vi "x410_test_fpga_with_ref.vi"() -> ()   [LabVIEW 2025]
doc: "this VI is the top level of the FPGA.\n\nsubVIs placed at this level:\nmust have fixed-sized arrays.\ncontaining a class input (control) must NOT be left unconnected.\n\nconditional symbols supported for ease-of-use in building variations of the image are documented in a comment section and should be kept up-to-date."
uses:
  <vilib>/Platform/TimedLoop/XDataNode/timing_clust.ctl
  <vilib>/Platform/TimedLoop/XDataNode/nitl_modes.ctl
  <vilib>/Platform/TimedLoop/XDataNode/wakeup.ctl
  Aqc_loop_states.ctl
  <vilib>/rvi/Emulation/niFpgaSctlEmulationGetInTimedLoop.vi
  <vilib>/rvi/Emulation/niFpgaEmulationReportErrorSimple.vi
  <vilib>/rvi/Emulation/niFpgaGetClockAttributes.vi
  <vilib>/rvi/Emulation/niFpgaCriticalErrorInLSC.vi
  <vilib>/rvi/Emulation/niFpgaProcessEmulError.vi
  <vilib>/rvi/interface/RandomDataEmulation/nirviRandomDataMultiElementFPGAFIFO.vi
  <instcachedir>/0/nirviRandomDataMultiElementFPGAFIFO_BE2FF10D3D6E420AB0291A02835C249E.lvgen/nirviRandomDataMultiElementFPGAFIFO_BE2FF10D3D6E420AB0291A02835C249E_001.vi
  <vilib>/rvi/interface/RandomDataEmulation/niFpgaRandomDataHandleErrors.vi
  <vilib>/Platform/TimedLoop/XDataNode/XDataNode.xnode
  <vilib>/rvi/DataTransferAndStorage/Container/XNode/niFpgaContainer.xnode
  <vilib>/rvi/interface/RandomDataEmulation/nirviRandomDataFpgaMultiElementTemplate.vi
  <instrlib>/niUSRP/Reference FPGA/Instruction Framework/niUSRP Reference FPGA v1.lvclass
  Reference FPGA/Rx DSP/niUSRP Rx DSP v2 FPGA.lvclass
  <instrlib>/niUSRP/Reference FPGA/Rx Core/niUSRP Rx Core v1 FPGA.lvclass
  <instrlib>/niUSRP/Reference FPGA/Sync/niUSRP Rx Core v1 FPGA/niUSRP Sync v1 FPGA.lvclass
  <instrlib>/niUSRP/Reference FPGA/Tx DSP/niUSRP Tx DSP v2 FPGA.lvclass
  <vilib>/Platform/TimedLoop/XDataNode/XDNodeRunTimeDep.lvlib
  <instrlib>/niUSRP/Reference FPGA/Stream Control/niUSRP Stream Control (DMA) v1 FPGA.lvclass
  <instrlib>/_niInstr/FIFO Register Bus/v1/FPGA/niInstr FIFO Register Bus v1 FPGA.lvclass
  <instrlib>/_niInstr/Instruction Framework/v1/FPGA/Collection Builder/Collection Builder.lvclass
  <instrlib>/niUSRP/Reference FPGA/Tx Core/niUSRP Tx Core v1 FPGA.lvclass
  <vilib>/rvi/FIFO/Fifo_Resource/nirvififoEmulationRead.vi
  <vilib>/rvi/FIFO/Fifo_Resource/nirvififoEmulationWrite.vi
  <vilib>/rvi/DataTransferAndStorage/Register/Emulation/niFpgaRegisterEmulation.vi
panel:
  in  "Record length":u16=4000 caption="Samples Per Trigger" min=1 step=1
  in  "Trigger Acquisition":bool
  in  "Acquisition running":bool
  out "fifo reg bus data 0":u64
  out "fifo reg bus status 0":u32
  in  "fifo reg bus ctrl 0":u32
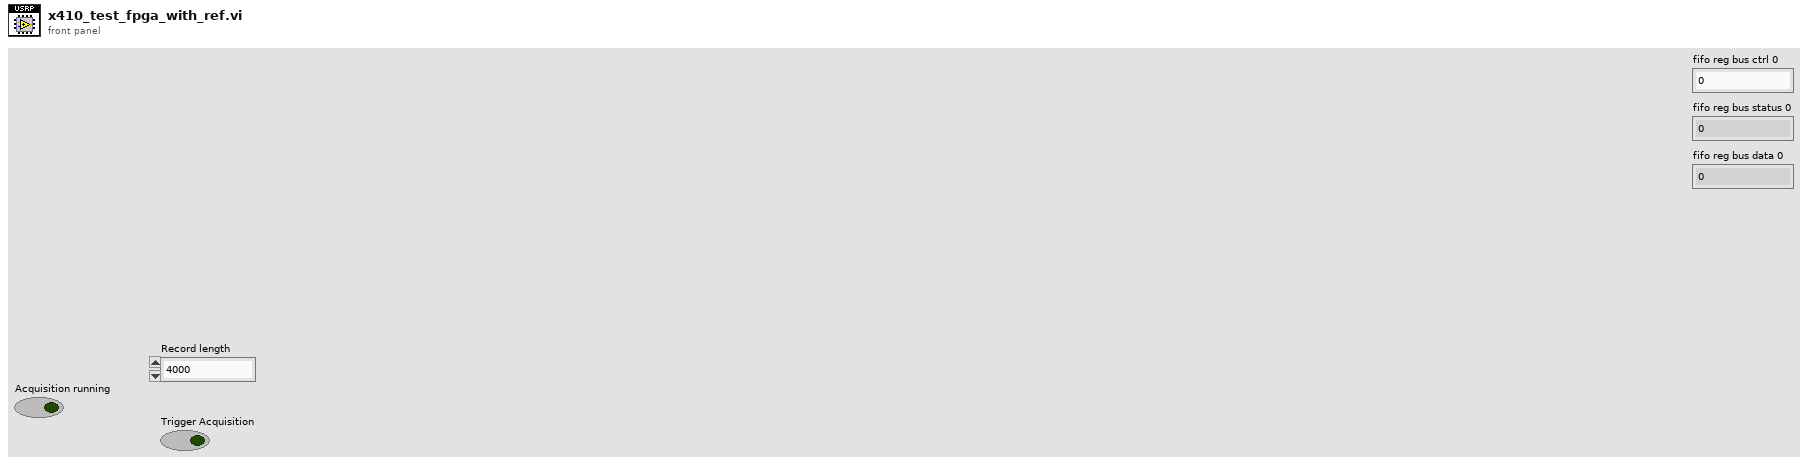
[diagram p1: front panel]
types:
  T1 = typedef "Aqc_loop_states.ctl" = enum8{"Wait for trigger", "Acquisition", "Send record length", "Wait for output", "Quiet period"}
  T2 = typedef "XDNodeRunTimeDep.lvlib/timing_clust.ctl" = cluster{"Expected End [f-1]":u64, "Actual End [f-1]":u64, "Finished Late? [f-1]":bool, "Expected End [i-1]":u64, "Actual End [i-1]":u64, "Finished Late? [i-1]":bool, "Expected Start [i]":u64, "Actual Start [i]":u64, "Expected Start [f]":u64, "Actual Start [f]":u64, "Source Name":string, "Structure Name":string, "Period":i64, "Deadline":i64, "Offset":i64, "Start":i64, "Priority":i32, "Timeout":i32, "Mode":T3, "Wakeup Reason":T4, "Error":errorcluster, "Source Type":string, "Secondary Source Type":string, "Global End Time":u64, "Global Start Time":u64, "Frame Duration":u64, "Iteration Duration":u64, "Assigned CPU":i32, "I/O Scan Engine Mode":u32}
  T3 = typedef "XDNodeRunTimeDep.lvlib/nitl_modes.ctl" = enum32{"No Change", "Process missed periods, maintain original phase", "Discard missed periods, maintain original phase", "Process missed periods, ignore original phase", "Discard missed periods, ignore original phase"}
  T4 = typedef "XDNodeRunTimeDep.lvlib/wakeup.ctl" = enum32{"Normal", "Aborted", "Asynchronous wakeup", "Timing source error", "Timed loop error", "Timeout"}
  T5 = typedef "niInstr DSP v1 Shared.lvlib/IQ Data.ctl" = cluster{"I":fxp<+/-,18,1>, "Q":fxp<+/-,18,1>, "overflow":bool}
  T6 = typedef "IQ-18bit-8element.ctl" = fxp<+/-,18,1>[]
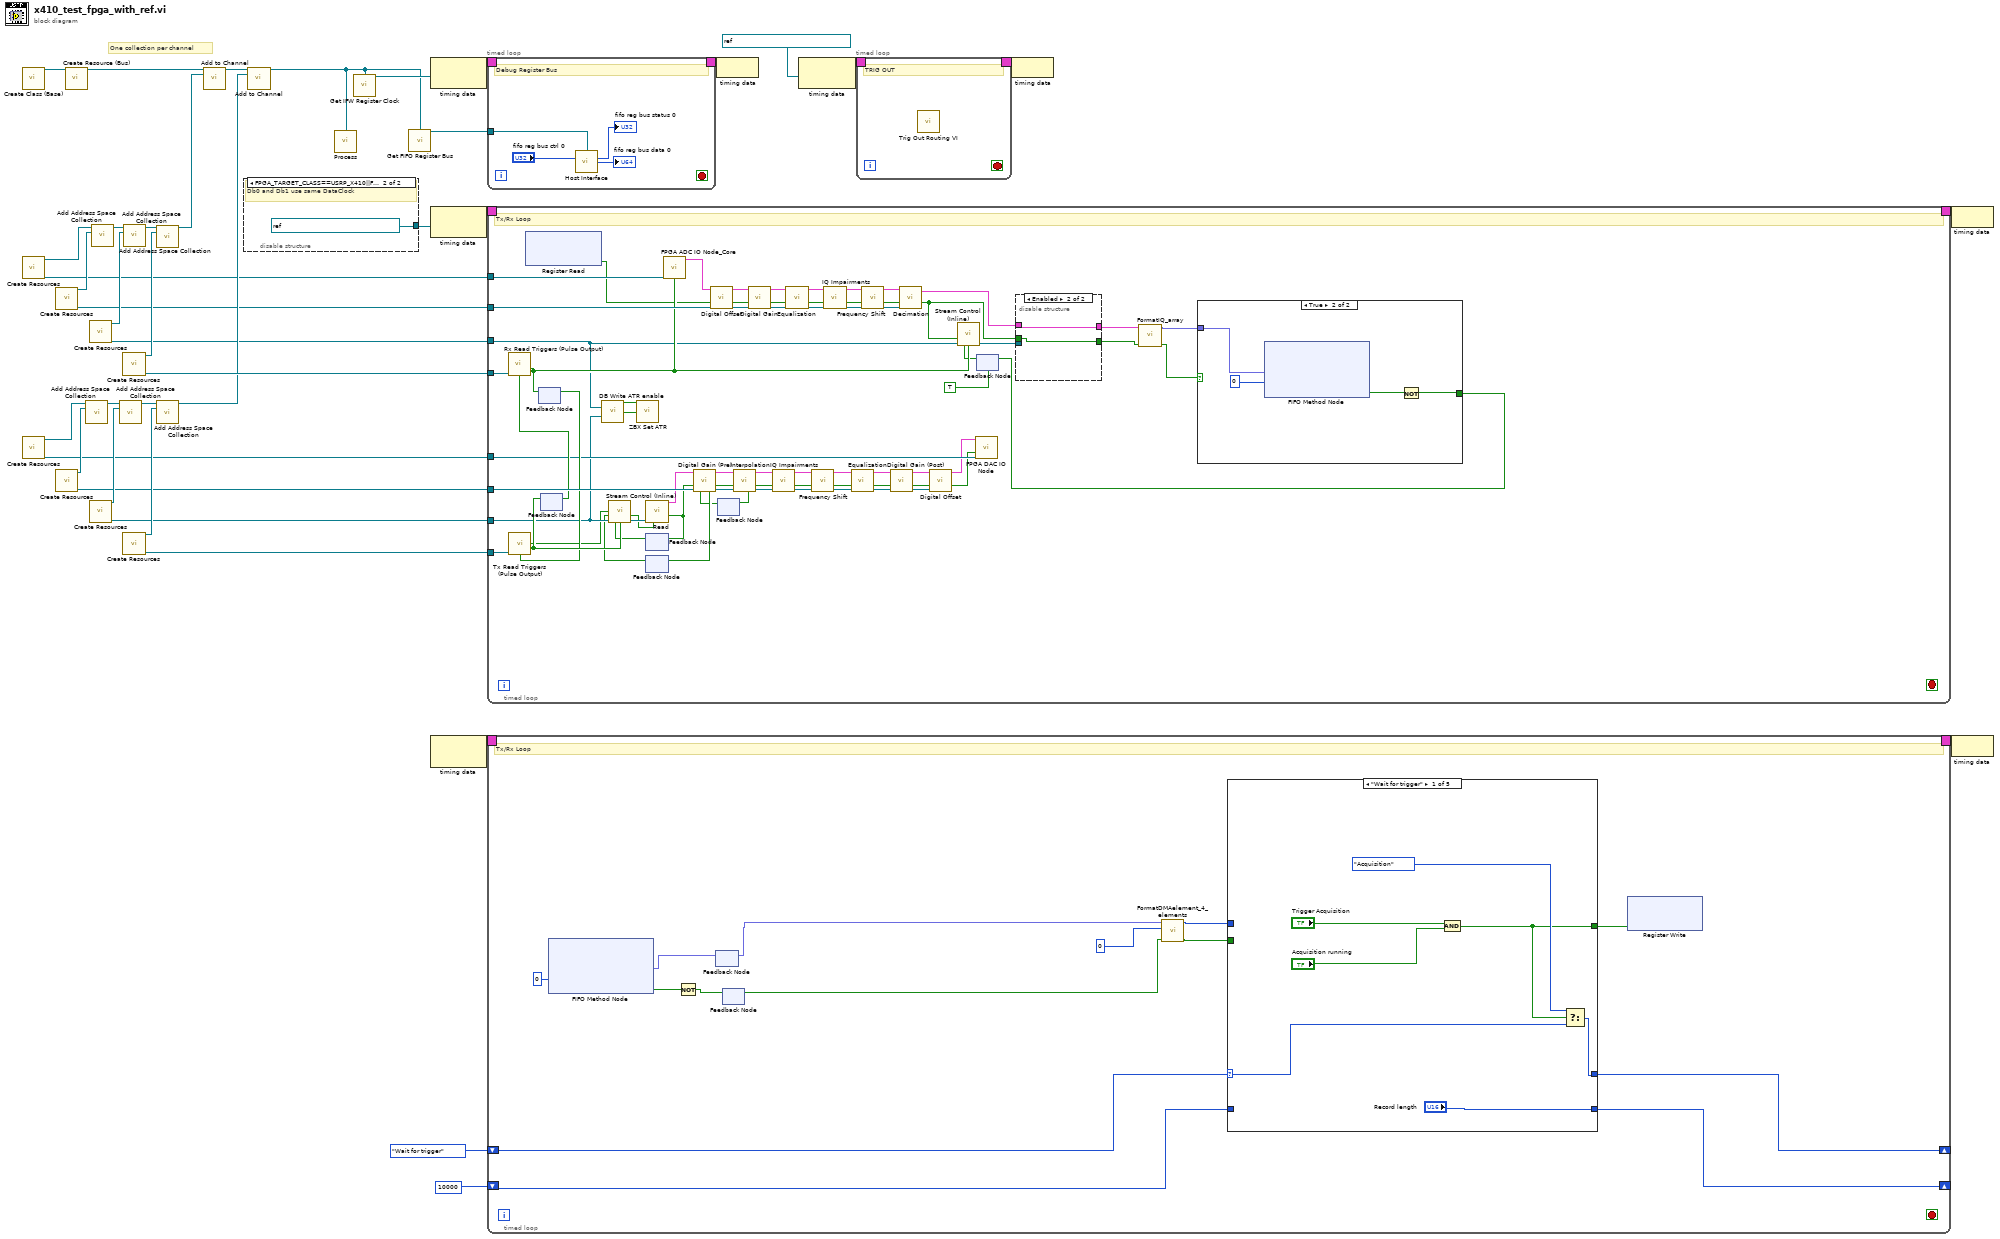
[diagram p0: block diagram]
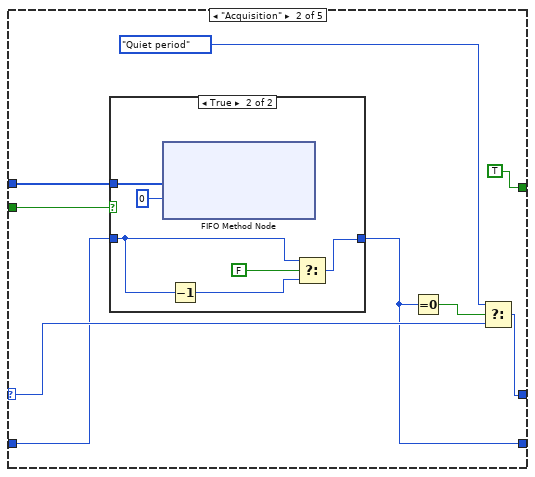
[diagram p2: hidden frame]
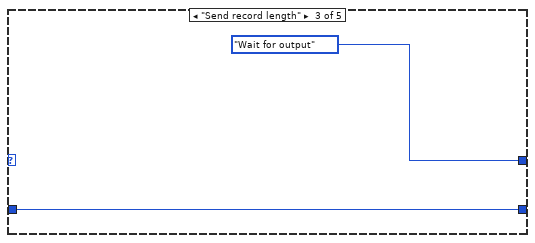
[diagram p4: hidden frame]
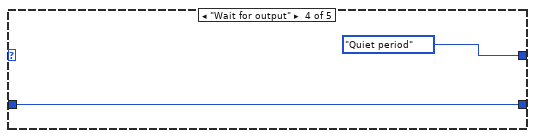
[diagram p5: hidden frame]
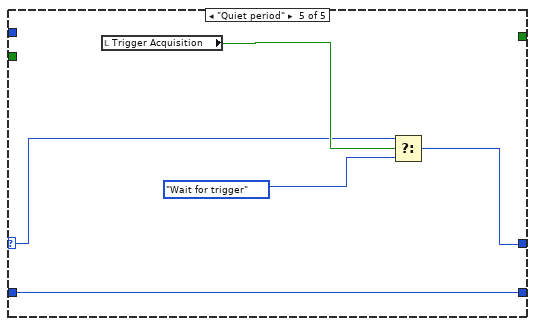
[diagram p6: hidden frame]
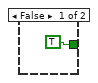
[diagram p7: hidden frame]
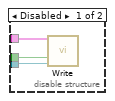
[diagram p8: hidden frame]
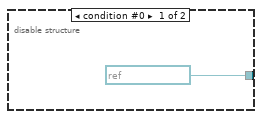
[diagram p9: hidden frame]
diagram:
  # "One collection per channel"
  n1 = call <instrlib>:"Create Class (Base).vi"() -> ("reference fpga"=w38:refnum<class "niUSRP Reference FPGA v1.lvclass">)  [unwired: 15 in]
  n2 = call <instrlib>:"Create Resources.vi"() -> ("channel collection builder"=w31:refnum<class "Collection Builder.lvclass">, "niVST Common Reference FPGA.lvclass"=w10:refnum<class "niUSRP Rx Core v1 FPGA.lvclass">)  [unwired: 14 in]
  n3 = call <instrlib>:"Create Resources.vi"() -> ("channel collection builder"=w23:refnum<class "Collection Builder.lvclass">, "niUSRP Tx Core"=w13:refnum<class "niUSRP Tx Core v1 FPGA.lvclass">)  [unwired: 14 in]
  n4 = call <instrlib>:"Create Resources.vi"() -> ("address space collection"=w35:refnum<class "Address Space Collection.lvclass">, "acq dsp session"=w5:refnum<class "niUSRP Rx DSP v2 FPGA.lvclass">)  [unwired: 14 in]
  n5 = call <instrlib>:"Create Resources.vi"() -> ("address space collection"=w22:refnum<class "Address Space Collection.lvclass">, "tx dsp"=w15:refnum<class "niUSRP Tx DSP v2 FPGA.lvclass">)  [unwired: 14 in]
  n6 = call-dynamic "Create Resource (Bus).vi"("reference fpga in"=w38) -> ("reference fpga out"=w34:refnum<class "niUSRP Reference FPGA v1.lvclass">)  [unwired: 14 in]
  n7 = call <instrlib>:"Add Address Space Collection.vi"("collection builder in"=w23, "address space collection"=w22) -> ("collection builder out"=w21:refnum<class "Collection Builder.lvclass">)  [unwired: 13 in]
  n8 = call <instrlib>:"Create Resources.vi"() -> ("address space collection"=w18:refnum<class "Address Space Collection.lvclass">, "stream session"=w12:refnum<class "niUSRP Stream Control (DMA) v1 FPGA.lvclass">)  [unwired: 14 in]
  n9 = call <instrlib>:"Create Resources.vi"() -> ("address space collection"=w25:refnum<class "Address Space Collection.lvclass">, "stream session"=w11:refnum<class "niUSRP Stream Control (DMA) v1 FPGA.lvclass">)  [unwired: 14 in]
  n10 = call <instrlib>:"Add Address Space Collection.vi"("collection builder in"=w31, "address space collection"=w35) -> ("collection builder out"=w33:refnum<class "Collection Builder.lvclass">)  [unwired: 13 in]
  n11 = call <instrlib>:"Add Address Space Collection.vi"("collection builder in"=w21, "address space collection"=w25) -> ("collection builder out"=w27:refnum<class "Collection Builder.lvclass">)  [unwired: 13 in]
  n12 = call <instrlib>:"Create Resources.vi"() -> ("address space collection"=w17:refnum<class "Address Space Collection.lvclass">, "stream control session"=w32:refnum<class "niUSRP Sync v1 FPGA.lvclass">)  [unwired: 14 in]
  n13 = call <instrlib>:"Create Resources.vi"() -> ("address space collection"=w24:refnum<class "Address Space Collection.lvclass">, "stream control session"=w14:refnum<class "niUSRP Sync v1 FPGA.lvclass">)  [unwired: 14 in]
  n14 = call <instrlib>:"Add Address Space Collection.vi"("collection builder in"=w33, "address space collection"=w18) -> ("collection builder out"=w30:refnum<class "Collection Builder.lvclass">)  [unwired: 13 in]
  n15 = call <instrlib>:"Add Address Space Collection.vi"("collection builder in"=w30, "address space collection"=w17) -> ("collection builder out"=w29:refnum<class "Collection Builder.lvclass">)  [unwired: 13 in]
  n16 = call <instrlib>:"Add Address Space Collection.vi"("collection builder in"=w27, "address space collection"=w24) -> ("collection builder out"=w26:refnum<class "Collection Builder.lvclass">)  [unwired: 13 in]
  n17 = call-dynamic "Add to Channel.vi"("reference fpga in"=w34, "collection builder in"=w29) -> ("reference fpga out"=w28:refnum<class "niUSRP Reference FPGA v1.lvclass">)  [unwired: 13 in]
  n18 = disable-structure shown="FPGA_TARGET_CLASS==USRP_X410||FPGA_TARGET_CLASS==USRP_X410__EMBEDDED____UNSUPPORTED" {
    disable-tunnel: [refnum<k21> "Data Clock" ("Source Name") refnum<k21> "Daughterboard 0\\Data Clock" ("Source Name")] -> w7
    frame condition #0 {
    }
    frame condition #1 (active) {
      # "Db0 and Db1 use same DataClock"
    }
  }
  n19 = call-dynamic "Add to Channel.vi"("reference fpga in"=w28, "collection builder in"=w26) -> ("reference fpga out"=w16:refnum<class "niUSRP Reference FPGA v1.lvclass">)  [unwired: 13 in]
  n20 = call <instrlib>:"Process.vi"("reference fpga"=w16) -> ()  [unwired: 15 in]
  n21 = call-dynamic "Get IFW Register Clock.vi"("reference fpga"=w16) -> ("ifw register clock"=w36:refnum<k21>)  [unwired: 14 in]
  n22 = call-dynamic "Get FIFO Register Bus.vi"("reference fpga"=w16) -> ("fifo register bus"=w37:refnum<class "niInstr FIFO Register Bus v1 FPGA.lvclass">)  [unwired: 14 in]
  n23 = node-c288 ("Input Node")(w36) -> (w40:T2)
  n24 = node-c288(w7) -> (w20:T2)
  n25 = node-c288() -> (w4:T2)  [unwired: 1 in]
  n26 = timed-loop {
    timing: w40 -> [_]
    timing-out: [_] -> w39
    tunnel: w37 -> [w43]
    stop <- _ stop-if-true
    # "Debug Register Bus"
    n27 = call <instrlib>:"Host Interface.vi"("fifo register bus"=w43, "fifo reg bus ctrl 0"="fifo reg bus ctrl 0") -> ("fifo reg bus status 0"=→"fifo reg bus status 0":u32, "fifo reg bus data 0"=→"fifo reg bus data 0":u64)  [unwired: 12 in]
  }
  n28 = timed-loop "Acquisition Loop" {
    timing: w20 -> [_]
    timing-out: [_] -> w19
    tunnel: w5 -> [w119]
    tunnel: w10 -> [w111]
    tunnel: w32 -> [w118]
    tunnel: w12 -> [w107]
    tunnel: w13 -> [w110]
    tunnel: w15 -> [w117]
    tunnel: w11 -> [w106]
    tunnel: w14 -> [w116]
    stop <- _ stop-if-true
    # "Tx/Rx Loop"
    n29 = xnode "Register Read"() -> ("Data"=w49:bool)  [unwired: 1 in, 1 out]
    n30 = feedback #1() -> (w112:bool)  [unwired: 1 in]
    n31 = call-dynamic "Tx Read Triggers (Pulse Output).vi"("niUSRP Sync"=w116, "external trigger"=w112) -> ("future trigger"=w105:bool, "output valid"=w115:bool)  [unwired: 10 in, 2 out]
    n32 = feedback #2() -> (w113:bool)  [unwired: 1 in]
    n33 = call-dynamic "Rx Read Triggers (Pulse Output).vi"("niUSRP Sync"=w118, "external trigger"=w113) -> ("output valid"=w114:bool)  [unwired: 11 in, 2 out]
    n34 = feedback-in #1(w114) -> ()
    n35 = feedback-in #2(w115) -> ()
    n36 = call <instrlib>:"DB Write ATR enable.vi"("stream session rx"=w107, "stream session tx"=w106) -> ("db 0"=w109:bool[], "db1"=w108:bool[])  [unwired: 12 in]
    n37 = call <instrlib>:"ZBX Set ATR.vi"("DB 1"=w108, "DB 0"=w109) -> ()  [unwired: 10 in]
    n38 = feedback #3() -> (w63:bool)  [unwired: 1 in]
    n39 = feedback #4() -> (w64:bool)  [unwired: 1 in]
    n40 = call <instrlib>:"Stream Control (Inline).vi"("future trigger"=w105, "input valid"=w64, "stream control"=w106, "ready for output"=w63, "trigger"=w115) -> ("stream"=w66:bool, "stream control"=w73:refnum<class "niUSRP Stream Control (DMA) v1 FPGA.lvclass">)  [unwired: 7 in, 2 out]
    n41 = call <instrlib>:"Read.vi"("stream control"=w73, "ready for output"=w66) -> ("data out"=w75:T5[], "output valid"=w65:bool)  [unwired: 11 in, 1 out]
    n42 = feedback-in #3(w65) -> ()
    n43 = call-dynamic "FPGA ADC IO Node_Core.vi"("rx core"=w111, "trigger"=w114) -> ("data"=w86:T5[])  [unwired: 10 in, 3 out]
    n44 = call-dynamic "Digital Offset.vi"("data in"=w86, "input valid"=w49, "acq in"=w119) -> ("data out"=w104:T5[], "output valid"=w103:bool, "acq out"=w102:refnum<class "niUSRP Rx DSP v2 FPGA.lvclass">)  [unwired: 9 in, 1 out]
    n45 = feedback #5() -> (w58:bool)  [unwired: 1 in]
    n46 = call-dynamic "Digital Gain (Pre).vi"("data in"=w75, "input valid"=w65, "gen in"=w117, "ready for output (T)"=w58) -> ("data out"=w60:T5[], "output valid"=w62:bool, "ready for input"=w74:bool, "gen out"=w61:refnum<class "niUSRP Tx DSP v2 FPGA.lvclass">)  [unwired: 8 in]
    n47 = feedback-in #4(w74) -> ()
    n48 = call-dynamic "Interpolation.vi"("data in"=w60, "input valid"=w62, "gen in"=w61) -> ("data out"=w84:T5[], "output valid"=w77:bool, "ready for input"=w59:bool, "gen out"=w76:refnum<class "niUSRP Tx DSP v2 FPGA.lvclass">)  [unwired: 9 in]
    n49 = feedback-in #5(w59) -> ()
    n50 = call-dynamic "Digital Gain.vi"("data in"=w104, "input valid"=w103, "acq in"=w102) -> ("data out"=w99:T5[], "output valid"=w100:bool, "acq out"=w101:refnum<class "niUSRP Rx DSP v2 FPGA.lvclass">)  [unwired: 9 in, 1 out]
    n51 = call-dynamic "IQ Impairments.vi"("data in"=w84, "input valid"=w77, "gen in"=w76) -> ("data out"=w72:T5[], "output valid"=w69:bool, "gen out"=w70:refnum<class "niUSRP Tx DSP v2 FPGA.lvclass">)  [unwired: 9 in, 1 out]
    n52 = call-dynamic "Equalization.vi"("data in"=w99, "input valid"=w100, "acq in"=w101) -> ("data out"=w98:T5[], "output valid"=w97:bool, "acq out"=w96:refnum<class "niUSRP Rx DSP v2 FPGA.lvclass">)  [unwired: 9 in, 1 out]
    n53 = call-dynamic "Frequency Shift.vi"("data in"=w72, "input valid"=w69, "gen in"=w70) -> ("data out"=w71:T5[], "output valid"=w68:bool, "gen out"=w67:refnum<class "niUSRP Tx DSP v2 FPGA.lvclass">)  [unwired: 9 in, 1 out]
    n54 = call-dynamic "IQ Impairments.vi"("data in"=w98, "input valid"=w97, "acq in"=w96) -> ("data out"=w94:T5[], "output valid"=w92:bool, "acq out"=w91:refnum<class "niUSRP Rx DSP v2 FPGA.lvclass">)  [unwired: 9 in, 1 out]
    n55 = call-dynamic "Equalization.vi"("data in"=w71, "input valid"=w68, "gen in"=w67) -> ("data out"=w83:T5[], "output valid"=w78:bool, "gen out"=w79:refnum<class "niUSRP Tx DSP v2 FPGA.lvclass">)  [unwired: 9 in, 1 out]
    n56 = call-dynamic "Frequency Shift.vi"("data in"=w94, "input valid"=w92, "acq in"=w91) -> ("data out"=w93:T5[], "output valid"=w89:bool, "acq out"=w90:refnum<class "niUSRP Rx DSP v2 FPGA.lvclass">)  [unwired: 9 in, 1 out]
    n57 = call-dynamic "Digital Gain (Post).vi"("data in"=w83, "input valid"=w78, "gen in"=w79) -> ("data out"=w82:T5[], "output valid"=w80:bool, "gen out"=w81:refnum<class "niUSRP Tx DSP v2 FPGA.lvclass">)  [unwired: 9 in, 1 out]
    n58 = call-dynamic "Decimation.vi"("data in"=w93, "input valid"=w89, "acq in"=w90) -> ("data out"=w87:T5[], "output valid"=w56:bool)  [unwired: 9 in, 2 out]
    n59 = call-dynamic "Digital Offset.vi"("data in"=w82, "input valid"=w80, "gen in"=w81) -> ("data out"=w57:T5[], "output valid"=w85:bool)  [unwired: 9 in, 2 out]
    n60 = call <instrlib>:"FPGA DAC IO Node.vi"("data"=w57, "input valid"=w85, "niUSRP Tx Core v1 FPGA.lvclass"=w110) -> ()  [unwired: 13 in]
    n61 = feedback #6(TRUE ("Timed Out?")) -> (w88:bool)
    n62 = call <instrlib>:"Stream Control (Inline).vi"("input valid"=w56, "stream control"=w107, "ready for output"=w88, "trigger"=w114) -> ("stream control"=w95:refnum<class "niUSRP Stream Control (DMA) v1 FPGA.lvclass">)  [unwired: 8 in, 3 out]
    n63 = disable-structure shown="Enabled" {
      disable-tunnel: w95 -> [w127 _]
      disable-tunnel: w56 -> [w126 w129]
      disable-tunnel: w87 -> [w125 w130]
      disable-tunnel: [_ w130] -> w55
      disable-tunnel: [_ w129] -> w54
      frame Disabled {
        n64 = call <instrlib>:"Write.vi"("data in"=w125, "input valid"=w126, "stream control"=w127) -> ("ready for input"=w128:bool)  [unwired: 11 in, 1 out]
      }
      frame Enabled {
      }
    }
    n65 = call "FormatIQ_array"("valid in"=w54, "data in"=w55) -> ("valid out"=w53:bool, "Array"=w52:T6)  [unwired: 8 in]
    n66 = case shown="True" w53 {
      tunnel: w52 -> [_ w123]
      tunnel: [TRUE ("Timed Out?") w121] -> w51
      frame False {
      }
      frame True {
        n67 = xnode ("FIFO Method Node")("Element"=w123, "Timeout"=0) -> ("Timed Out?"=w122:bool)  [unwired: 1 in, 1 out]
        n68 = Not(x=w122) -> (.not. x?=w121:bool)
      }
    }
    n69 = feedback-in #6(w51) -> ()
  }
  n70 = timed-loop "Acquisition Loop" {
    timing: w4 -> [_]
    timing-out: [_] -> w3
    shift-right: [w142] -> _
    shift-left: u16 10000 ("Record length") -> [w140]
    shift-right: [w143] -> _
    shift-left: Aqc_loop_states."Wait for trigger" ("loop states") -> [w141]
    stop <- _ stop-if-true
    # "Tx/Rx Loop"
    n71 = xnode ("FIFO Method Node")("Timeout"=0) -> ("Element"=w135:fxp<+/-,18,1>[], "Timed Out?"=w138:bool)  [unwired: 1 in, 1 out]
    n72 = Not(x=w138) -> (.not. x?=w137:bool)
    n73 = feedback #7() -> (w134:fxp<+/-,18,1>[])  [unwired: 1 in]
    n74 = feedback-in #7(w135) -> ()
    n75 = feedback-in #8(w137) -> ()
    n76 = feedback #8() -> (w136:bool)  [unwired: 1 in]
    n77 = call "FormatDMAelement_4_elements.vi"("valid in"=w136, "factor"=u16 0, "Array"=w134) -> ("valid out"=w144:bool, "Values"=w145:u64[])  [unwired: 7 in]
    n78 = case shown="\"Wait for trigger\"" w141 {
      selector: w141 -> [w153 w162 _ _ w175]
      tunnel: w140 -> [_ w159 w171 w173 w176]
      tunnel: [w152 w161 Aqc_loop_states."Wait for output" ("loop states") Aqc_loop_states."Quiet period" ("loop states") w177] -> w143
      tunnel: ["Record length" w156 w171 w173 w176] -> w142
      tunnel: w145 -> [_ w157 _ _ _]
      tunnel: w144 -> [_ w158 _ _ _]
      tunnel: [w147 TRUE _ _ _] -> w133
      frame "Wait for trigger" {
        n79 = And(x="Trigger Acquisition", y="Acquisition running") -> (x .and. y?=w147:bool)
        n80 = Select(t=Aqc_loop_states."Acquisition" ("loop states"), s=w147, f=w153) -> (s? t:f=w152:T1)
      }
      frame "Acquisition" {
        n81 = case shown="True" w158 {
          tunnel: w157 -> [_ w169]
          tunnel: [w163 w167] -> w156
          tunnel: w159 -> [w163 w165]
          frame False {
          }
          frame True {
            n82 = xnode ("FIFO Method Node")("Element"=w169, "Timeout"=0) -> ()  [unwired: 1 in, 2 out]
            n83 = Decrement(x=w165) -> (x-1=w166:u16)
            n84 = Select(t=w165, s=FALSE, f=w166) -> (s? t:f=w167:u16)
          }
        }
        n85 = Equal To 0?(x=w156) -> (x = 0?=w160:bool)
        n86 = Select(t=Aqc_loop_states."Quiet period" ("loop states"), s=w160, f=w162) -> (s? t:f=w161:T1)
      }
      frame "Send record length" {
      }
      frame "Wait for output" {
      }
      frame "Quiet period" {
        n87 = local read "Trigger Acquisition"() -> (w178:bool)
        n88 = Select(t=w175, s=w178, f=Aqc_loop_states."Wait for trigger" ("loop states")) -> (s? t:f=w177:T1)
      }
    }
    n89 = xnode "Register Write"("Data"=w133) -> ()  [unwired: 1 in, 1 out]
  }
  n90 = node-c288(w39) -> ()
  n91 = node-c288 ("Input Node")(refnum<k21> "Daughterboard 0\\Data Clock" ("Source Name")) -> (w9:T2)
  n92 = timed-loop {
    timing: w9 -> [_]
    timing-out: [_] -> w8
    stop <- _ stop-if-true
    # "TRIG OUT"
    n93 = call <instrlib>:"Trig Out Routing VI.vi"() -> ()  [unwired: 16 in]
  }
  n94 = node-c288(w8) -> ()
  n95 = node-c288(w19) -> ()
  n96 = node-c288(w3) -> ()
